vi "InitDGObj and HW.vi"(4 "error out":errorcluster, 6 "DGNr":i32, 7 "BME_DG_System in":refnum<class "BME_DG_System.lvclass">) -> (0 "error IO":errorcluster, 3 "BME_DG_System Out":refnum<class "BME_DG_System.lvclass">)   [LabVIEW 2009, in "POLARIS BME DG.lvlib" / "BME_DG_System.lvclass"]
uses:
  BME_DG_System.lvclass
  BME_DG_Base/BME_DG_Base.lvclass
  BME_DG_G08/BME_DG_G08.lvclass
  BME_DG_G02/BME_DG_G02.lvclass
  BME_DG_G05P2/BME_DG_G05P2.lvclass
  BME_DG_G05/BME_DG_G05.lvclass
  BME_DG_System.lvclass/BME_DG_System.ctl
  POLARIS BME DG.lvlib
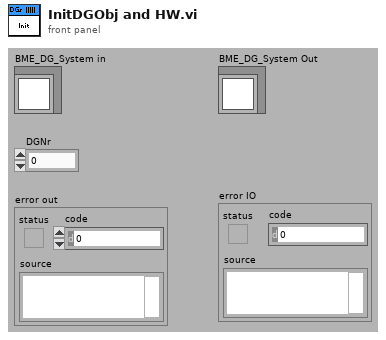
[diagram p1: front panel]
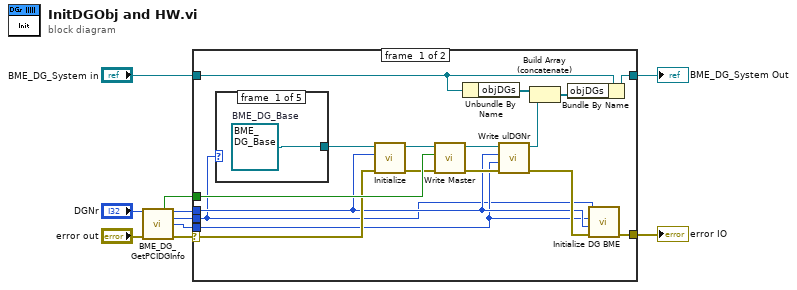
[diagram p0: block diagram]
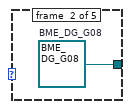
[diagram p2: hidden frame]
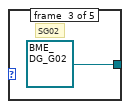
[diagram p3: hidden frame]
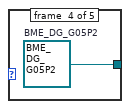
[diagram p4: hidden frame]
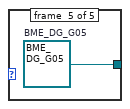
[diagram p5: hidden frame]
diagram:
  n1 = call "BME_DG_GetPCIDGInfo.vi"("DG_Number in"="DGNr", "error in (no error)"="error out") -> ("Master"=w6:bool, "DG_Number out"=w7:i32, "DG_Product"=w2:i32, "SlotNumber"=w8:i32, "error out"=w3:errorcluster)  [unwired: 9 in]
  n2 = case shown="No Error" w3 {
    selector: w3 -> [w18 w33]
    tunnel: w2 -> [w11 _]
    tunnel: [w27 w34] -> w4
    tunnel: "BME_DG_System in" -> [w25 w34]
    tunnel: w6 -> [w21 _]
    tunnel: w7 -> [w13 _]
    tunnel: w8 -> [w12 _]
    tunnel: [w15 w33] -> w10
    frame #0 {
      n3 = case shown="20, 40, 43" w11 {
        tunnel: [w28 w29 refnum<class "BME_DG_G02.lvclass"> refnum ("BME_DG_G02.lvclass") w31 w32] -> w19
        frame #0 {
          w28 = refnum<class "BME_DG_Base.lvclass"> refnum  # BME_DG_Base
        }
        frame #1 {
          w29 = refnum<class "BME_DG_G08.lvclass"> refnum  # BME_DG_G08
        }
        frame #2 {
          # "SG02"
        }
        frame #3 {
          w31 = refnum<class "BME_DG_G05P2.lvclass"> refnum  # BME_DG_G05P2
        }
        frame #4 {
          w32 = refnum<class "BME_DG_G05.lvclass"> refnum  # BME_DG_G05
          # "G05"
        }
      }
      n4 = call-dynamic "Initialize.vi"("error in (no error)"=w18, "DG Nr"=w13, "BME_DG_Base in"=w19) -> ("error out"=w17:errorcluster, "BME_DG_Base out"=w16:refnum<class "BME_DG_Base.lvclass">)  [unwired: 7 in]
      n5 = call-dynamic "Write Master.vi"("error in (no error)"=w17, "Master?"=w21, "BME_DG_Base in"=w16) -> ("error out"=w23:errorcluster, "BME_DG_Base out"=w22:refnum<class "BME_DG_Base.lvclass">)  [unwired: 7 in]
      n6 = Unbundle By Name(w25) -> ("objDGs"=w24:refnum<class "BME_DG_Base.lvclass">[])
      n7 = call-dynamic "Write ulDGNr.vi"("error in (no error)"=w23, "ulSlotNr"=w12, "ulDGNr"=w13, "BME_DG_Base in"=w22) -> ("error out"=w14:errorcluster, "BME_DG_Base out"=w20:refnum<class "BME_DG_Base.lvclass">)  [unwired: 6 in]
      n8 = Build Array (concatenate)(w24, w20) -> (w26:refnum<class "BME_DG_Base.lvclass">[])
      n9 = Bundle By Name(cluster=w25, "objDGs"=w26) -> (w27:refnum<class "BME_DG_System.lvclass">)
      n10 = call "Initialize DG BME.vi"("error in (no error)"=w14, "DG Number"=w13, "Slot Number"=w12, "DG Product"=w11) -> ("error out"=w15:errorcluster)  [unwired: 7 in]
    }
    frame #1 {
    }
  }
  "error IO" <- w10
  "BME_DG_System Out" <- w4
